vi "OnValueChange_System.vi"(8 "error in (no error)":errorcluster, 9 "Value":bool, 11 "SnakeGame in":refnum<class "SnakeGame.lvclass">) -> (0 "error out":errorcluster, 3 "SnakeGame out":refnum<class "SnakeGame.lvclass">)   [LabVIEW 2019, in "RT_Game.lvlib" / "SnakeGame.lvclass"]
uses:
  SnakeGame.lvclass
  C:/Users/FreshBob/Dropbox/VIs/myRIO_GameConsole/RT/RT_Game/Game/Game.lvclass
  SnakeGame.lvclass/SnakeGame.ctl
  Menu/States.ctl
  Game/Game.lvclass/Game.ctl
  Game/Write State.vi
  Game/Game.lvclass
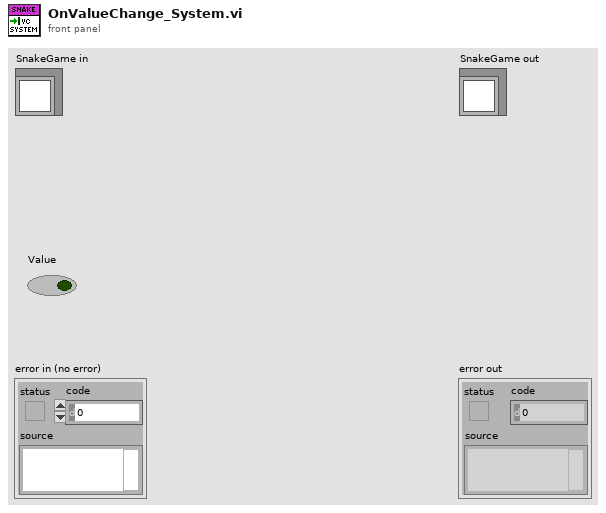
[diagram p1: front panel]
types:
  T1 = typedef "RT_Game.lvlib/Game.lvclass/States.ctl" = enum16{"Init", "Restart", "Menu", "Game", "Resume", "ToggleSingleplayer", "LoadNextGame", "ExitToMenu", "NewHighscore", "GameOver", "SlideOut", "FadeToMenu", "StartFadeToMenu"}
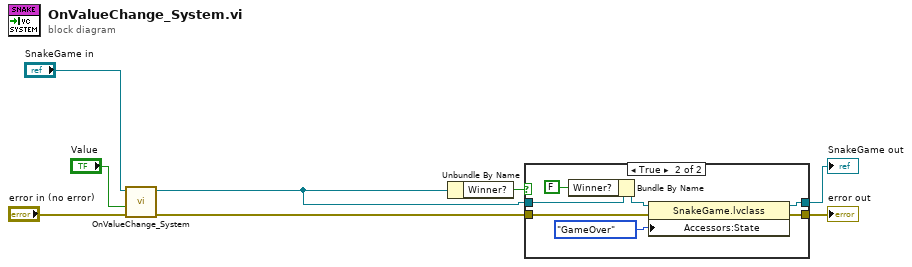
[diagram p0: block diagram]
diagram:
  n1 = call-parent "OnValueChange_System.vi"("error in (no error)"="error in (no error)", "Value"="Value", "Game in"="SnakeGame in") -> ("error out"=w8:errorcluster, "Game out"=w2:refnum<class "SnakeGame.lvclass">)  [unwired: 7 in]
  n2 = Unbundle By Name(w2) -> ("Winner?"=w1:bool)
  n3 = case shown="True" w1 {
    tunnel: w8 -> [w9 w17]
    tunnel: [w9 w16] -> w4
    tunnel: [w10 w15] -> w3
    tunnel: w2 -> [w10 w14]
    frame False {
    }
    frame True {
      n4 = Bundle By Name(cluster=w14, "Winner?"=FALSE) -> (w12:refnum<class "SnakeGame.lvclass">)
      n5 = property class="SnakeGame.lvclass"(reference=w12, error in=w17, "Accessors:State"=States."GameOver" ("State")) -> (reference out=w15:refnum<class "SnakeGame.lvclass">, error out=w16:errorcluster)
    }
  }
  "error out" <- w4
  "SnakeGame out" <- w3
